vi "Throw Test Error.vi"(8 "error in (no error)":errorcluster, 11 "Route Manager in":refnum<class "Route Manager.lvclass">) -> (0 "error out":errorcluster, 3 "Route Manager out":refnum<class "Route Manager.lvclass">)   [LabVIEW 2015, in "Route Manager.lvclass"]
uses:
  Route Manager.lvclass
  Route Manager.lvclass/Route Manager.ctl
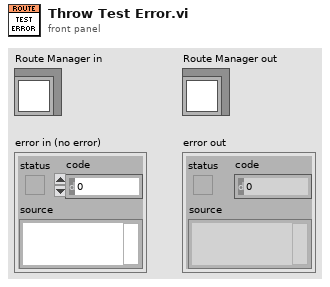
[diagram p1: front panel]
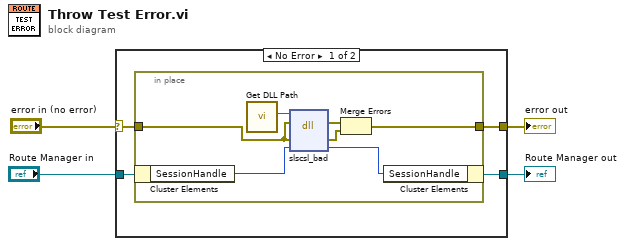
[diagram p0: block diagram]
diagram:
  n1 = case shown="No Error" "error in (no error)" {
    selector: "error in (no error)" -> [w6 w17]
    tunnel: [w5 w17] -> w3
    tunnel: [w7 w16] -> w1
    tunnel: "Route Manager in" -> [w8 w16]
    frame No Error {
      n2 = in-place {
        in-place-border: w6 -> [w12]
        in-place-border: [w9] -> w5
        n3 = in-place-cluster #1(w8) -> ("SessionHandle"=w13:u64)
        n4 = call "Get DLL Path.vi"() -> ("slscsl DLL Path"=w15:path)  [unwired: 11 in]
        n5 = dll-call lib="?" fn="slscsl_bad"(path in=w15, error in=w12, "errorCluster"=w12, "sessionHandle"=w13) -> (error out=w10:errorcluster, "errorCluster"=w11:errorcluster, "sessionHandle"=w14:u64)  [unwired: 2 in, 1 out]
        n6 = Merge Errors(w10, w11) -> (w9:errorcluster)
        n7 = in-place-cluster #1("SessionHandle"=w14) -> (w7:refnum<class "Route Manager.lvclass">)
      }
    }
    frame Error {
    }
  }
  "error out" <- w3
  "Route Manager out" <- w1
